vi "Analog Input Status.vi"(7 "Unit Address (1)":i16=1, 8 "error in (no error)":errorcluster {"code" format="%.0x"}, 10 "Item To Read (0: Input 1 Error Status)":u16(ring) items=["Input 1 Error Status", "Input 1 Open Loop Status", "Input 2 Error Status", "Input 2 Open Loop Status", "Input 3 Error Status"], 11 "VISA resource name":refnum<visa-resource-name>) -> (0 "error out":errorcluster {"code" format="%.0x"}, 2 "Value":i32, 3 "VISA resource name out":refnum<visa-resource-name>)   [LabVIEW 2010]
doc: "This VI returns base instrument informations."
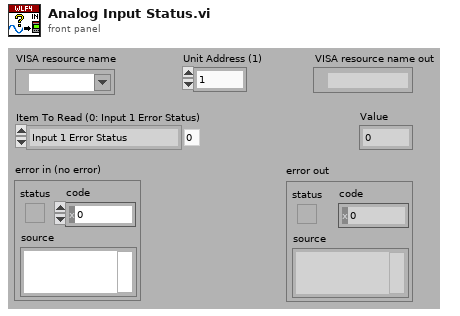
[diagram p1: front panel]
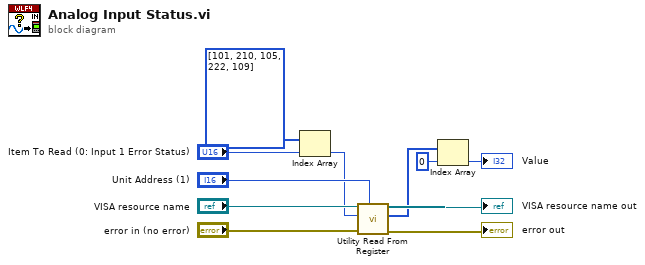
[diagram p0: block diagram]
diagram:
  n1 = Index Array(array=i32[] [101, 210, 105, 222, 109], index="Item To Read (0: Input 1 Error Status)") -> (element=w5:i32)
  n2 = call "Utility Read From Register.vi"("Unit Address (1)"="Unit Address (1)", "error in (no error)"="error in (no error)", "Register Address (0)"=w5, "VISA resource name"="VISA resource name") -> ("error out"=→"error out":errorcluster, "Data"=w2:i16[], "VISA resource name out"=→"VISA resource name out":refnum<visa-resource-name>)  [unwired: 5 in]
  n3 = Index Array(array=w2, index=0) -> (element=→"Value":i16)
